vi "micro_2.vi"(6 "result":string, 7 "Type":string, 8 "err":bool, 9 "SN":string, 10 "version":string, 11 "PN":string) -> (3 "Chaîne":string)   [LabVIEW 2020]
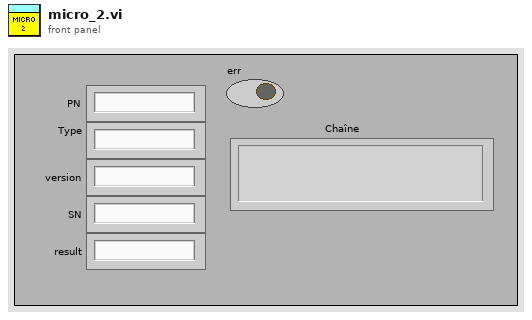
[diagram p1: front panel]
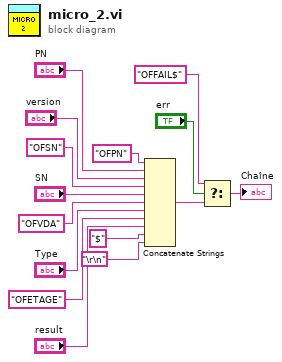
[diagram p0: block diagram]
diagram:
  n1 = Concatenate Strings("OFPN" ("chaîne"), "PN", "version", "OFSN" ("chaîne"), "SN", "OFVDA" ("chaîne"), "Type", "OFETAGE" ("chaîne"), "result", "$" ("chaîne"), "\r\n") -> (w2:string)
  n2 = Select(t="OFFAIL$", s="err", f=w2) -> (s? t:f=→"Chaîne":string)
